vi "Configure NF Monitor Spectrum Bandwidth.vi"(0 "VISA resource name":refnum<visa-resource-name>, 5 "Resolution Bandwidth (0 Hz)":dbl format="%^#_6g", 7 "Video Bandwidth (0 Hz)":dbl format="%^#_6g", 9 "Video to Resolution Bandwidth Ratio (1)":dbl=1.0 format="%^#_6g", 11 "error in (no error)":errorcluster) -> (4 "VISA resource name out":refnum<visa-resource-name>, 15 "error out":errorcluster)   [LabVIEW 2014, in "Agilent ESA PSA Series.lvlib"]
doc: "Configures the bandwidth settings of the Monitor Spectrum measurement of the Noise Figure personality.\n\n<B>Note:</B> \n\nThis VI is only valid in Noise Figure personality. Use <B>Switch Personality</B> VI to switch to Noise Figure before calling this VI."
uses:
  Agilent ESA PSA Series.lvlib
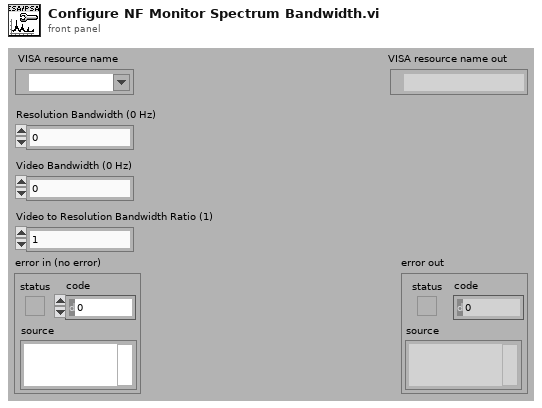
[diagram p1: front panel]
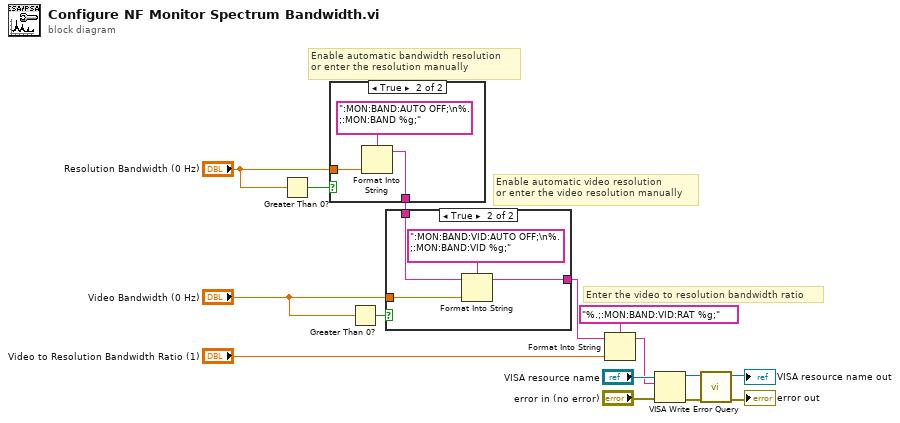
[diagram p0: block diagram]
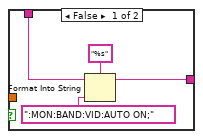
[diagram p2: hidden frame]
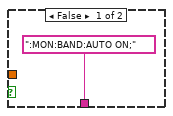
[diagram p3: hidden frame]
diagram:
  # "Enter the video to resolution bandwidth ratio"
  # "Enable automatic video resolution\nor enter the video resolution manually"
  # "Enable automatic bandwidth resolution\nor enter the resolution manually"
  n1 = Greater Than 0?(x="Resolution Bandwidth (0 Hz)") -> (x > 0?=w9:bool)
  n2 = case shown="True" w9 {
    tunnel: "Resolution Bandwidth (0 Hz)" -> [_ w19]
    tunnel: [":MON:BAND:AUTO ON;" w17] -> w5
    frame False {
    }
    frame True {
      n3 = Format Into String(format string=":MON:BAND:AUTO OFF;\n%.;:MON:BAND %g;", w19) -> (resulting string=w17:string)  [unwired: 2 in, 1 out]
    }
  }
  n4 = Greater Than 0?(x="Video Bandwidth (0 Hz)") -> (x > 0?=w7:bool)
  n5 = case shown="True" w7 {
    tunnel: "Video Bandwidth (0 Hz)" -> [_ w27]
    tunnel: [w20 w25] -> w4
    tunnel: w5 -> [w23 w24]
    frame False {
      n6 = Format Into String(format string="%s", initial string=w23, ":MON:BAND:VID:AUTO ON;") -> (resulting string=w20:string)  [unwired: 1 in, 1 out]
    }
    frame True {
      n7 = Format Into String(format string=":MON:BAND:VID:AUTO OFF;\n%.;:MON:BAND:VID %g;", initial string=w24, w27) -> (resulting string=w25:string)  [unwired: 1 in, 1 out]
    }
  }
  n8 = Format Into String(format string="%.;:MON:BAND:VID:RAT %g;", initial string=w4, "Video to Resolution Bandwidth Ratio (1)") -> (resulting string=w1:string)  [unwired: 1 in, 1 out]
  n9 = VISA Write(VISA resource name="VISA resource name", write buffer=w1, error in (no error)="error in (no error)") -> (VISA resource name out=w13:refnum<visa-resource-name>, error out=w12:errorcluster)  [unwired: 1 out]
  n10 = call "Error Query.vi"("error in (no error)"=w12, "VISA resource name"=w13) -> ("error out"=→"error out":errorcluster, "VISA resource name out"=→"VISA resource name out":refnum<visa-resource-name>)  [unwired: 6 in, 2 out]
